vi "Sign Data Example Algorithm.vi"(11 "data":variant) -> (3 "signature":string)   [LabVIEW 2016]
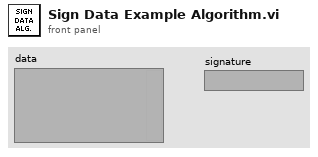
[diagram p1: front panel]
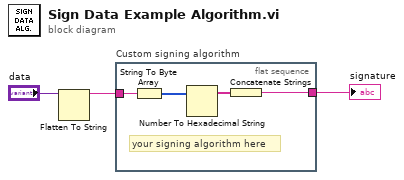
[diagram p0: block diagram]
diagram:
  n1 = Flatten To String(anything="data") -> (data string=w1:string)  [unwired: 3 in, 2 out]
  n2 = flat-sequence "Custom signing algorithm" {
    tunnel: [w5] -> w3
    tunnel: w1 -> [w4]
    frame #0 {
      # "your signing algorithm here"
      n3 = String To Byte Array(string=w4) -> (unsigned byte array=w7:u8[])
      n4 = Number To Hexadecimal String(2:w7) -> (0:w6:string[])  [unwired: 1 in]
      n5 = Concatenate Strings(w6) -> (w5:string)
    }
  }
  "signature" <- w3
